vi "AutofocusOptions.vi"() -> ()   [LabVIEW 2019]
panel:
  out "output string":string
  out "value":dbl
  out "Last Z, mean and standard deviation:":string
  in  "Stop":bool
  in  "Path to Text File":path=path "C:/Users/TTUHEP/Documents/LabVIEW/GantryPrograms/Configs/SensorPositions.txt"
  out "error out":errorcluster
  out "Best Z value":string
  in  "Filter Type":T1(ring)=enum."Sobel"
  in  "error in (no error)":errorcluster
  in  "SpeedZ (mm/s)":dbl=10.0
  in  "SpeedXY (mm/s)":dbl=100.0
  in  "Z":dbl
  in  "Y":dbl
  in  "X":dbl
  in  "ControlType":T2(ring)=enum."Option 3" caption="Operation Mode"
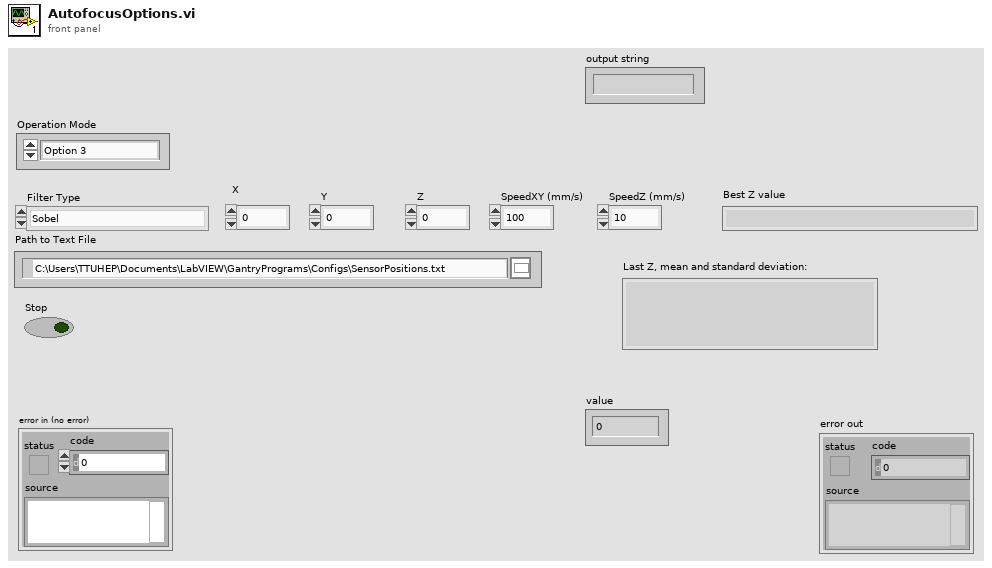
[diagram p1: front panel]
types:
  T1 = enum16{"Convolution", "Differentiation", "Gradient", "Prewitt", "Roberts", "Sigma", "Sobel"}
  T2 = enum16{"Single Point Measurement", "Text File", "Option 3"}
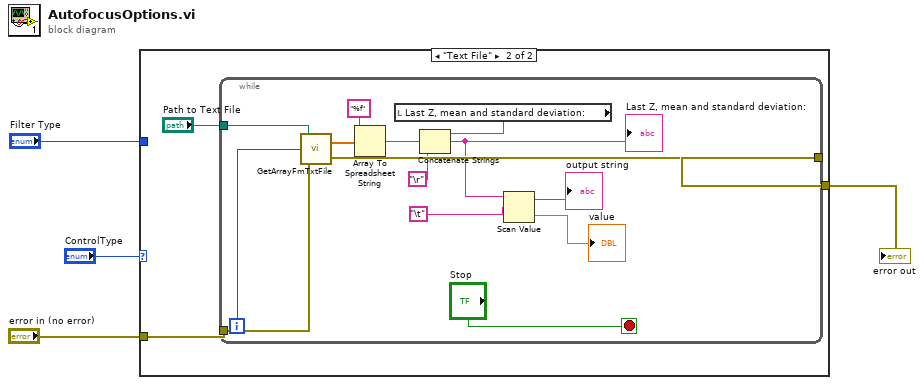
[diagram p0: block diagram]
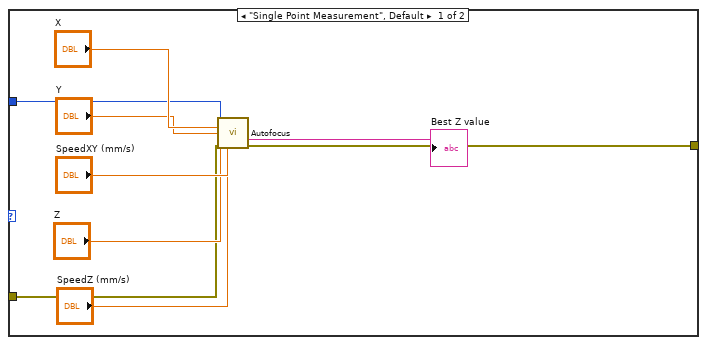
[diagram p2: hidden frame]
diagram:
  n1 = case shown="\"Text File\"" "ControlType" {
    tunnel: "error in (no error)" -> [w8 w15]
    tunnel: "Filter Type" -> [w7 _]
    tunnel: [w5 w14] -> w1
    frame "Single Point Measurement", Default {
      n2 = call "Autofocus.vi"("Filter Type"=w7, "SpeedXY (mm/s)"="SpeedXY (mm/s)", "X"="X", "Y"="Y", "Z"="Z", "error in (no error)"=w8, "SpeedZ (mm/s)"="SpeedZ (mm/s)") -> ("Best Z value"=→"Best Z value":string, "error out"=w5:errorcluster)  [unwired: 7 in]
    }
    frame "Text File" {
      n3 = while {
        tunnel: "Path to Text File" -> [w30]
        tunnel: w15 -> [w28]
        tunnel: [w27] -> w14
        i -> [w29]
        stop <- "Stop" stop-if-true
        n4 = call "GetArrayFmTxtFile.vi"("error in"=w28, "LineNo."=w29, "TextFile"=w30) -> ("error out"=w27:errorcluster, "Array"=w22:dbl[])
        n5 = Array To Spreadsheet String(array=w22, 3:"%f" ("format string")) -> (spreadsheet string=w21:string)  [unwired: 1 in]
        n6 = local read "Last Z, mean and standard deviation:"() -> (w23:string)
        n7 = Concatenate Strings(w23, w21, "\r") -> (w20:string)
        "Last Z, mean and standard deviation:" <- w20
        n8 = Scan Value(string=w20, format string="\t") -> (output string=→"output string":string, value=→"value":dbl)  [unwired: 1 in]
      }
    }
  }
  "error out" <- w1
